vi "复杂反馈节点.vi"() -> ()   [LabVIEW 2010]
panel:
  out "result":dbl
  out "result":dbl
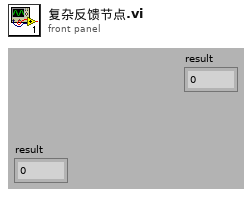
[diagram p1: front panel]
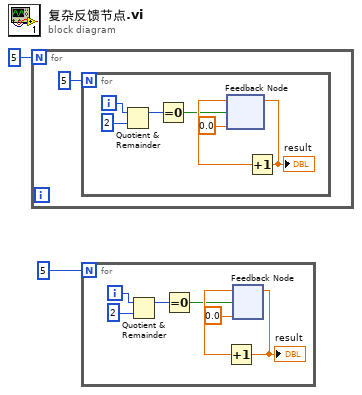
[diagram p0: block diagram]
diagram:
  n1 = for {
    N: 5 -> [_]
    n2 = for {
      N: 5 -> [_]
      i -> [w4]
      n3 = Quotient & Remainder(x=w4, y=2) -> (x-y*floor(x/y)=w6:i32)  [unwired: 1 out]
      n4 = Equal To 0?(x=w6) -> (x = 0?=w5:bool)
      n5 = feedback #1(0.0) -> (w9:dbl)
      n6 = Increment(x=w9) -> (x+1=w10:dbl)
      "result" <- w10
      n7 = feedback-in #1(w10, w5) -> ()
    }
  }
  n8 = for {
    N: 5 -> [_]
    i -> [w12]
    n9 = Quotient & Remainder(x=w12, y=2) -> (x-y*floor(x/y)=w13:i32)  [unwired: 1 out]
    n10 = Equal To 0?(x=w13) -> (x = 0?=w11:bool)
    n11 = feedback #2(0.0) -> (w16:dbl)
    n12 = Increment(x=w16) -> (x+1=w17:dbl)
    "result" <- w17
    n13 = feedback-in #2(w17, w11) -> ()
  }
